vi "ResolveHostRoot.vi"(8 "error in (no error)":errorcluster, 10 "Application:Kind":T1, 11 "HostApplicationPath":path) -> (0 "error out":errorcluster, 3 "HostRoot":path)   [LabVIEW 2026, in "Lumberjack.lvlib"]
doc: "Resolve the host root that empty or relative log paths are computed against (SRS-LMBR-064). If HostApplicationPath is supplied, use it. Otherwise, when running as a built application (Application.Kind = Run Time System), return error 5000 (host application path required), since defaulting to the executable folder is often read-only under UAC; when running in the development system, fall back to Application Directory. Never derives a path from a Lumberjack VI's own location (no Current VI's Path), so paths stay correct inside a .lvlibp"
uses:
  Lumberjack.lvlib
  TypeDefs/HostAppKind.ctl
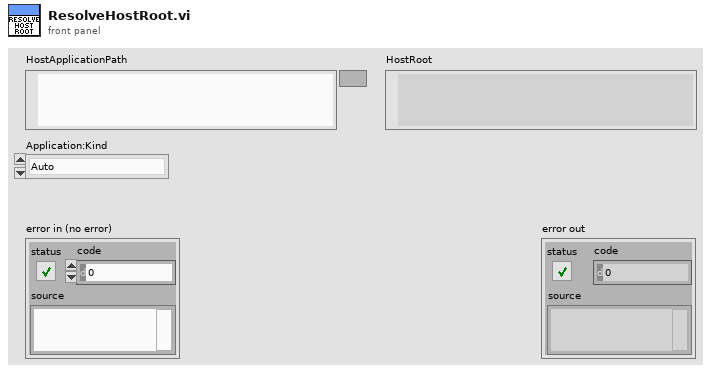
[diagram p1: front panel]
types:
  T1 = typedef "Lumberjack.lvlib/HostAppKind.ctl" = enum32{"Auto", "Development System", "Run Time System"}
  T2 = enum32{"invalid app kind", "Development System", "Run Time System", "Student Edition", "Embedded LabVIEW", "Evaluation", "Custom"}
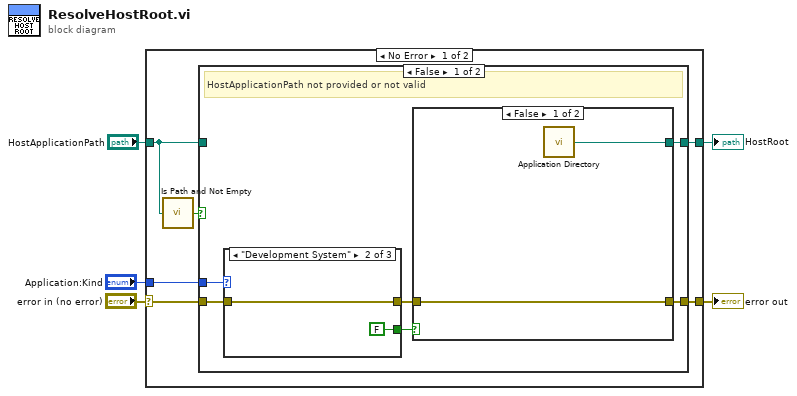
[diagram p0: block diagram]
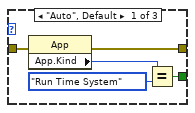
[diagram p2: hidden frame]
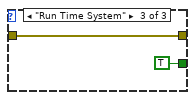
[diagram p3: hidden frame]
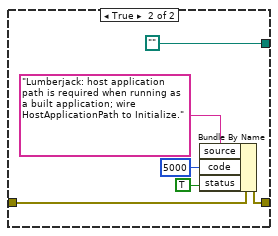
[diagram p4: hidden frame]
diagram:
  n1 = case shown="No Error" "error in (no error)" {
    selector: "error in (no error)" -> [w7 w38]
    tunnel: [w10 w38] -> w5
    tunnel: "HostApplicationPath" -> [w9 w37]
    tunnel: [w8 w37] -> w3
    tunnel: "Application:Kind" -> [w6 _]
    frame No Error {
      n2 = call <vilib>:"Is Path and Not Empty.vi"("path"=w9) -> ("Is Path and Not Empty?"=w11:bool)  [unwired: 4 in]
      n3 = case shown="False" w11 {
        tunnel: w7 -> [w16 w36]
        tunnel: [w17 w36] -> w10
        tunnel: w9 -> [_ w35]
        tunnel: [w13 w35] -> w8
        tunnel: w6 -> [w14 _]
        frame False {
          # "HostApplicationPath not provided or not valid"
          n4 = case shown="\"Development System\"" w14 {
            tunnel: w16 -> [w22 w24 w26]
            tunnel: [w21 w24 w26] -> w15
            tunnel: [w18 FALSE TRUE] -> w12
            frame "Auto", Default {
              n5 = property class="App"(error in=w22) -> (error out=w21:errorcluster, "App.Kind"=w20:T2)  [unwired: 1 in, 1 out]
              n6 = Equal?(x=w20, y=T2."Run Time System" ("Application:Kind")) -> (x = y?=w18:bool)
            }
            frame "Development System" {
            }
            frame "Run Time System" {
            }
          }
          n7 = case shown="False" w12 {
            tunnel: w15 -> [w28 w34]
            tunnel: [w28 w33] -> w17
            tunnel: [w27 path ""] -> w13
            frame False {
              n8 = call <vilib>:"Application Directory.vi"() -> ("Application Directory"=w27:path)
            }
            frame True {
              n9 = Bundle By Name(cluster=w34, "source"="Lumberjack: host application path is required when running as a built application; wire HostApplicationPath to Initialize.", "code"=5000, "status"=TRUE) -> (w33:errorcluster)
            }
          }
        }
        frame True {
          # "HostApplicationPath provided and valid"
        }
      }
    }
    frame Error {
    }
  }
  "error out" <- w5
  "HostRoot" <- w3
